vi "UpdateStates.vi"(8 "error in (no error)":errorcluster, 11 "DataPacker in":refnum<class "DataPacker.lvclass">) -> (0 "error out":errorcluster, 1 "Connection Attempt":u32, 2 "Frontend Status":string, 3 "DataPacker out":refnum<class "DataPacker.lvclass">, 4 "MIDAS Port":u16, 5 "MIDAS Addresss":string, 7 "Enum":T1)   [LabVIEW 2018, in "feGEM DataPacker.lvlib"]
uses:
  feGEM DataPacker.lvlib
  StateMachineTypeDef.ctl
  DataPacker.lvclass
  GlobalVariables/Set_And_Get_Enum.ctl
  DataPacker.lvclass/DataPacker.ctl
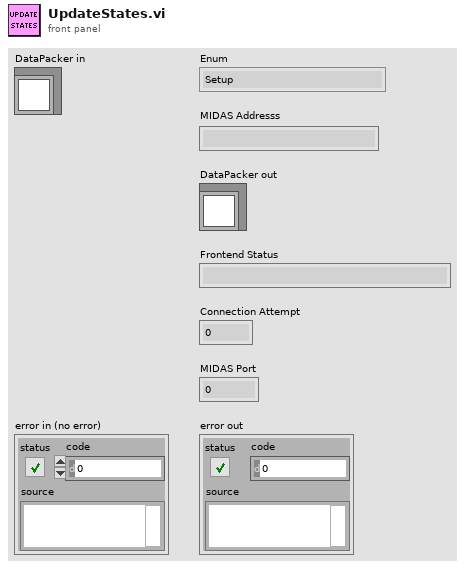
[diagram p1: front panel]
types:
  T1 = typedef "feGEM DataPacker.lvlib/StateMachineTypeDef.ctl" = enum16{"Setup", "Setup SSH", "Connect To Midas", "Get And Set Event Size", "Re-initialise", "Update status", "BundleDataInQueue", "SerializeBundle", "SendData", "Shutdown", "HandleErrorStates", "Wait"}
  T2 = typedef "feGEM DataPacker.lvlib/Set_And_Get_Enum.ctl" = enum16{"Set", "Get"}
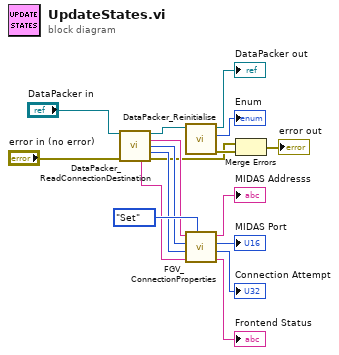
[diagram p0: block diagram]
diagram:
  n1 = call "DataPacker_ReadConnectionDestination.vi"("DataPacker in"="DataPacker in", "error in (no error)"="error in (no error)") -> ("DataPacker out"=w11:refnum<class "DataPacker.lvclass">, "MIDAS Addresss"=w9:string, "MIDAS Port"=w8:u16, "Connection Attempt"=w10:u32, "Frontend Status"=w12:string, "error out"=w1:errorcluster)  [unwired: 8 in]
  n2 = call "DataPacker_Reinitialise.vi"("DataPacker in"=w11) -> ("error out"=w3:errorcluster, "Next State"=→"Enum":T1, "DataPacker out"=→"DataPacker out":refnum<class "DataPacker.lvclass">)  [unwired: 8 in]
  n3 = call "FGV_ConnectionProperties.vi"("Enum"=Set_And_Get_Enum."Set", "Frontend Status in"=w12, "Connection Attempt in"=w10, "MIDAS Port in"=w8, "MIDAS Addresss in"=w9) -> ("Frontend Status out"=→"Frontend Status":string, "Connection Attempt out"=→"Connection Attempt":u32, "MIDAS Port out"=→"MIDAS Port":u16, "MIDAS Addresss out"=→"MIDAS Addresss":string)  [unwired: 3 in]
  n4 = Merge Errors(w1, w3) -> (→"error out":errorcluster)
